vi "Sandbox 2 - Add VI to lvlib.vi"(8 "error in":errorcluster) -> (0 "error out":errorcluster)   [LabVIEW 2021]
doc: "Sandbox"
panel:
  out "VI Path (rn)":path
  # "Development\ncontrols/indicators useful for development and testing, but which are not outputs of the VI"
  # "Input\nInputs to the VI"
  # "Output\nOutputs of the VI"
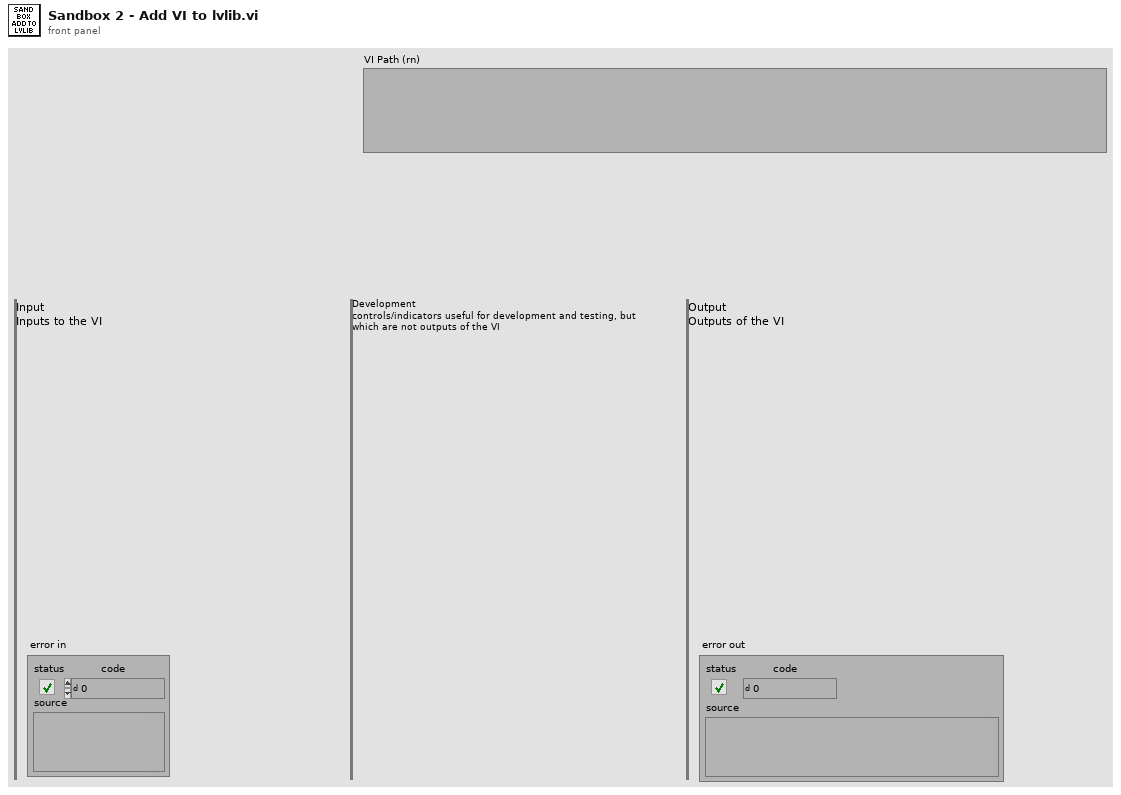
[diagram p1: front panel]
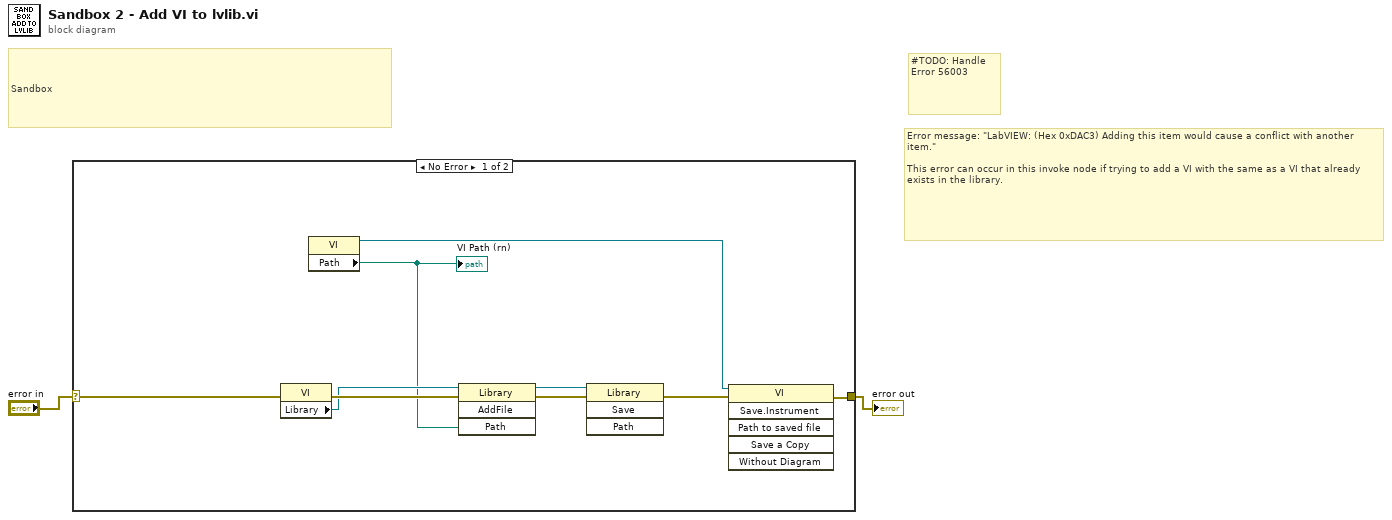
[diagram p0: block diagram]
diagram:
  # "Error message: \"LabVIEW: (Hex 0xDAC3) Adding this item would cause a conflict with another item.\"\n\nThis error can occur in this invoke node if trying to add a VI with the same as a VI that already exists in the library."
  # "#TODO: Handle \nError 56003"
  # "Sandbox"
  n1 = case shown="No Error" "error in" {
    selector: "error in" -> [w11 w12]
    tunnel: [w10 w12] -> w1
    frame No Error {
      n2 = property class="VI"(error in=w11) -> (error out=w9:errorcluster, "Library"=w8:refnum<vi>)  [unwired: 1 in, 1 out]
      n3 = property class="VI"() -> (reference out=w3:refnum<vi>, "Path"=w4:path)  [unwired: 2 in, 1 out]
      "VI Path (rn)" <- w4
      n4 = invoke class="Library" method="AddFile"(reference=w8, error in=w9, "Path"=w4) -> (reference out=w5:refnum<vi>, error out=w7:errorcluster)  [unwired: 1 in, 2 out]
      n5 = invoke class="Library" method="Save"(reference=w5, error in=w7) -> (error out=w6:errorcluster)  [unwired: 2 in, 3 out]
      n6 = invoke class="VI" method="Save.Instrument"(reference=w3, error in=w6) -> (error out=w10:errorcluster)  [unwired: 4 in, 5 out]
    }
    frame Error {
    }
  }
  "error out" <- w1
